vi "Get Item Depth & @ Locations.vi"(11 "Menu Item Description":string) -> (0 "Levels":string[](array[string]), 1 "@ Locations":cluster{"Array":i32[]}, 3 "Depth":i32)   [LabVIEW 2019]
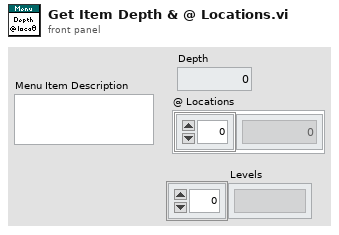
[diagram p1: front panel]
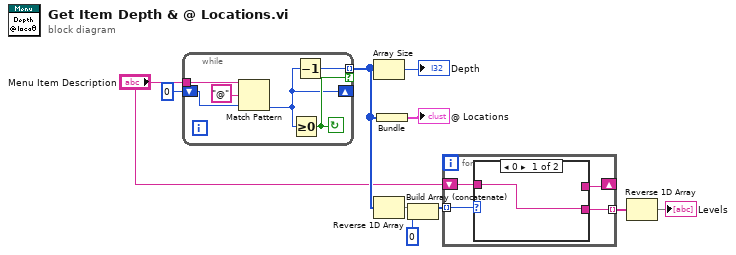
[diagram p0: block diagram]
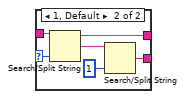
[diagram p2: hidden frame]
diagram:
  n1 = while {
    tunnel: "Menu Item Description" -> [w13]
    shift-right: [w12] -> _
    shift-left: 0 ("offset past token") -> [w14]
    tunnel: [w11] -> w7 mode=indexing if=w16
    stop <- w16 continue-if-true
    n2 = Match Pattern(string=w13, regular expression="@", offset (0)=w14) -> (offset past match=w12:i32)  [unwired: 3 out]
    n3 = Greater Or Equal To 0?(x=w12) -> (x >= 0?=w16:bool)
    n4 = Decrement(x=w12) -> (x-1=w11:i32)
  }
  n5 = Array Size(array=w7) -> (size(s)=→"Depth":i32)
  n6 = Reverse 1D Array(array=w7) -> (reversed array=w5:i32[])
  n7 = Bundle(w7) -> (→"@ Locations":cluster{i32[]})  [unwired: 1 in]
  n8 = Build Array (concatenate)(w5, 0) -> (w3:i32[])
  n9 = for {
    tunnel: w3 -> [w19] mode=indexing
    shift-right: [w18] -> _
    shift-left: "Menu Item Description" -> [w20]
    tunnel: [w17] -> w4 mode=indexing
    n10 = case shown="0" w19 {
      selector: w19 -> [_ w26]
      tunnel: w20 -> [w21 w27]
      tunnel: [_ w25] -> w18
      tunnel: [w21 w23] -> w17
      frame 0 {
      }
      frame 1, Default {
        n11 = Search/Split String(string=w27, offset (0)=w26) -> (substring before match=w25:string, match + rest of string=w24:string)  [unwired: 1 in, 1 out]
        n12 = Search/Split String(string=w24, offset (0)=1) -> (match + rest of string=w23:string)  [unwired: 1 in, 2 out]
      }
    }
  }
  n13 = Reverse 1D Array(array=w4) -> (reversed array=→"Levels":string[])
